vi "Register Instance.vi"(6 "Base Class (LabVIEW Object)":refnum<class>, 7 "Object Instance":refnum<data-value>, 8 "error in (no error)":errorcluster, 11 "Lookup Service in":refnum<data-value>) -> (0 "error out":errorcluster, 3 "Lookup Service out":refnum<data-value>)   [LabVIEW 2014, in "LVCOOOP.lvlib" / "Lookup API.lvlib" / "Lookup Service.lvclass"]
doc: "Associate an object instance with the specified base class."
uses:
  Lookup Service.lvclass
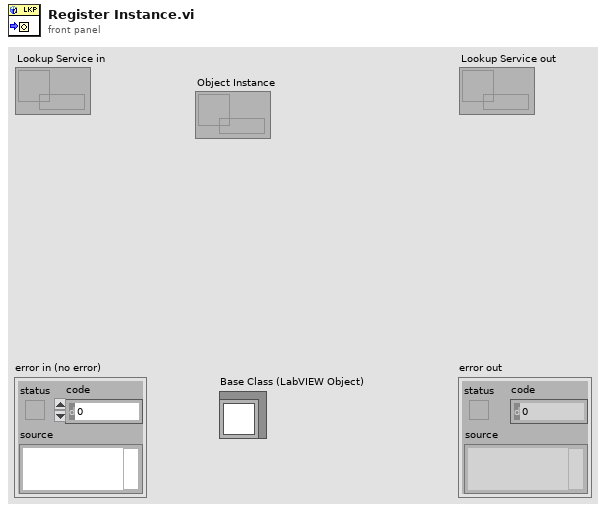
[diagram p1: front panel]
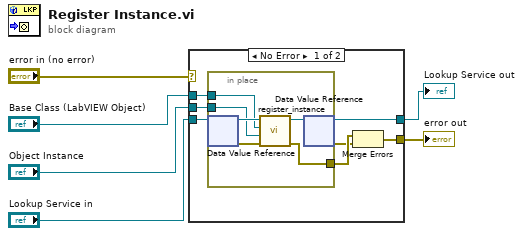
[diagram p0: block diagram]
diagram:
  n1 = case shown="No Error" "error in (no error)" {
    selector: "error in (no error)" -> [_ w20]
    tunnel: "Base Class (LabVIEW Object)" -> [w13 _]
    tunnel: "Lookup Service in" -> [w10 w21]
    tunnel: [w9 w21] -> w3
    tunnel: [w8 w20] -> w2
    tunnel: "Object Instance" -> [w7 _]
    frame No Error {
      n2 = in-place {
        in-place-border: w13 -> [w17]
        in-place-border: [w14] -> w12
        in-place-border: w7 -> [w16]
        n3 = in-place-dvr #1(w10) -> (w19:refnum<class "Lookup Service.lvclass">, w15:errorcluster)
        n4 = call-dynamic "register_instance.vi"("error in (no error)"=w15, "Object Instance"=w16, "Base Class (LabVIEW Object)"=w17, "Lookup Service in"=w19) -> ("error out"=w14:errorcluster, "Lookup Service out"=w18:refnum<class "Lookup Service.lvclass">)  [unwired: 6 in]
        n5 = in-place-dvr #1(w18) -> (w9:refnum<data-value>, w11:errorcluster)
      }
      n6 = Merge Errors(w12, w11) -> (w8:errorcluster)
    }
    frame Error {
    }
  }
  "error out" <- w2
  "Lookup Service out" <- w3
